vi "Report Status Changes.vi"(5 "Seq Name":string, 6 "Loop Data in":T1, 7 "VolatusAPI":refnum<class "VolatusAPI.lvclass">, 9 "Previous Late":bool, 10 "Previous Duration":i64, 11 "Sequence in":refnum<class "Sequence.lvclass">) -> (4 "Loop Data":T1)   [LabVIEW 2023, in "VolatusSeq.lvlib" / "Sequence.lvclass"]
uses:
  Sequence.lvclass
  Volatus/VolatusAPI/VolatusAPI.lvclass
  Loop Data.ctl
  Volatus/MessageQ/MessageQ.lvclass
  Sequence Time.ctl
  Sequence Status.ctl
  Sequence.lvclass/Sequence.ctl
  Volatus/MessageQ/MessageQ.lvclass/MessageQ.ctl
  VolatusSeq.lvlib
  State/State.lvclass
  VolatusSeqConfig/Debug Flags.ctl
  VolatusSeqConfig/VolatusSeqConfig.lvlib
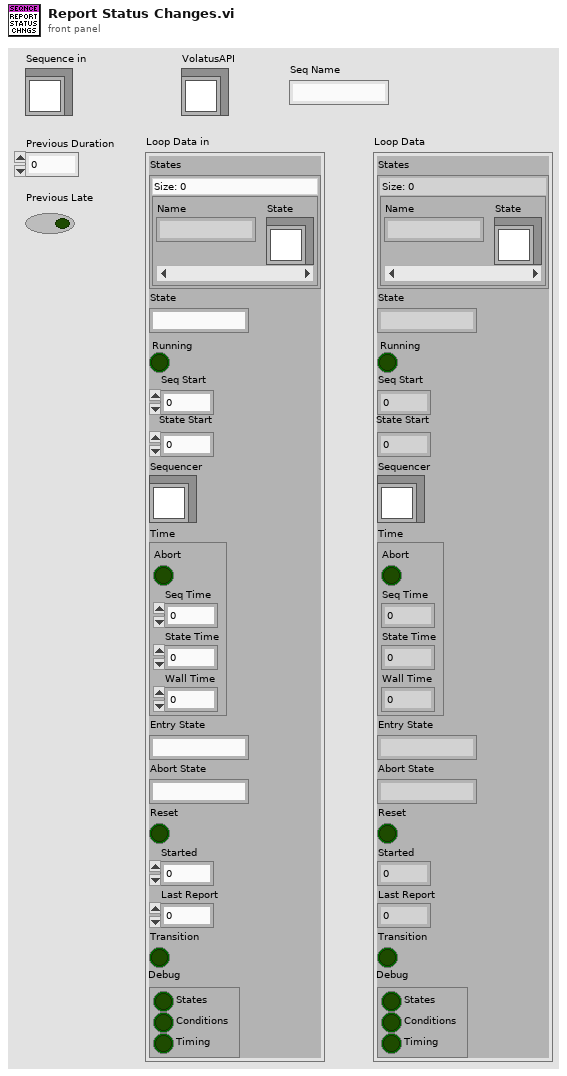
[diagram p1: front panel]
types:
  T1 = typedef "VolatusSeq.lvlib/Sequence.lvclass/Loop Data.ctl" = cluster{"States":map{string, refnum<class "State.lvclass">}, "State":string, "Running":bool, "Seq Start":dbl, "State Start":dbl, "Sequencer":refnum<class "MessageQ.lvclass">, "Time":T2, "Entry State":string, "Abort State":string, "Reset":bool, "Started":dbl, "Last Report":dbl, "Transition":bool, "Debug":T3}
  T2 = typedef "VolatusSeq.lvlib/Sequence Time.ctl" = cluster{"Abort":bool, "Seq Time":dbl, "State Time":dbl, "Wall Time":dbl}
  T3 = typedef "VolatusSeqConfig.lvlib/Debug Flags.ctl" = cluster{"States":bool, "Conditions":bool, "Timing":bool}
  T4 = typedef "VolatusSeq.lvlib/Sequence Status.ctl" = cluster{"Name":string, "State":string, "Time":T2, "Running":bool, "Start Time":dbl, "Previous Duration":i64, "Previous Late":bool}
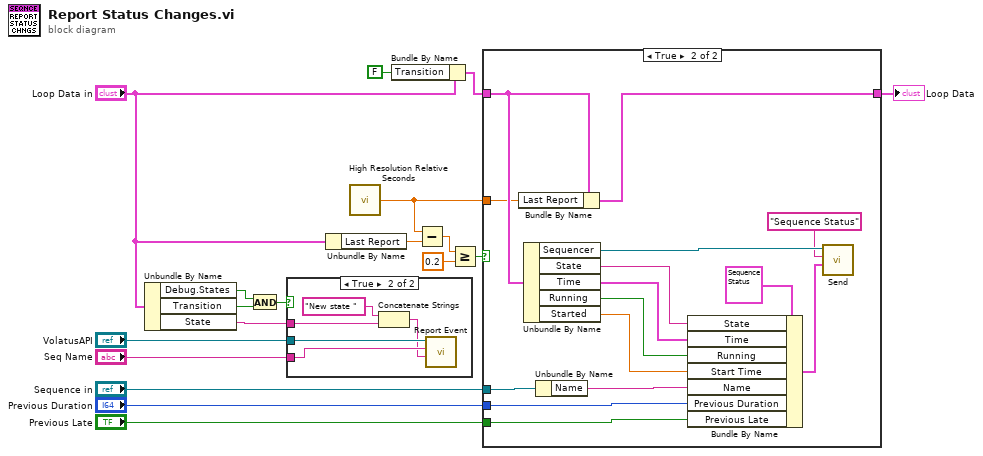
[diagram p0: block diagram]
diagram:
  n1 = Unbundle By Name("Loop Data in") -> ("Debug.States"=w5:bool, "Transition"=w6:bool, "State"=w3:string)
  n2 = And(x=w5, y=w6) -> (x .and. y?=w4:bool)
  n3 = case shown="True" w4 {
    tunnel: w3 -> [_ w20]
    tunnel: "VolatusAPI" -> [_ w23]
    tunnel: "Seq Name" -> [_ w22]
    frame False {
    }
    frame True {
      n4 = Concatenate Strings("New state ", w20) -> (w19:string)
      n5 = call "Report Event.vi"("Message"=w19, "Context"=w22, "VolatusAPI in"=w23) -> ()  [unwired: 7 in, 2 out]
    }
  }
  n6 = Unbundle By Name("Loop Data in") -> ("Last Report"=w15:dbl)
  n7 = call <vilib>:"High Resolution Relative Seconds.vi"() -> ("relative seconds"=w10:dbl)
  n8 = Bundle By Name(cluster="Loop Data in", "Transition"=FALSE) -> (w8:T1)
  n9 = Subtract(x=w10, y=w15) -> (x-y=w14:dbl)
  n10 = Greater Or Equal?(x=w14, y=0.2) -> (x >= y?=w12:bool)
  n11 = case shown="True" w12 {
    tunnel: "Sequence in" -> [_ w39]
    tunnel: "Previous Duration" -> [_ w29]
    tunnel: "Previous Late" -> [_ w28]
    tunnel: w8 -> [w24 w27]
    tunnel: [w24 w26] -> w11
    tunnel: w10 -> [_ w25]
    frame False {
    }
    frame True {
      n12 = Bundle By Name(cluster=w27, "Last Report"=w25) -> (w26:T1)
      n13 = Unbundle By Name(w27) -> ("Sequencer"=w34:refnum<class "MessageQ.lvclass">, "State"=w36:string, "Time"=w35:T2, "Running"=w31:bool, "Started"=w30:dbl)
      n14 = Unbundle By Name(w39) -> ("Name"=w37:string)
      n15 = Bundle By Name(cluster=T4 {"Name"="", "State"="", "Time"={"Abort"=FALSE, "Seq Time"=0.0, "State Time"=0.0, "Wall Time"=0.0}, "Running"=FALSE, "Start Time"=0.0, "Previous Duration"=0, "Previous Late"=FALSE} ("Sequence Status"), "State"=w36, "Time"=w35, "Running"=w31, "Start Time"=w30, "Name"=w37, "Previous Duration"=w29, "Previous Late"=w28) -> (w33:T4)
      n16 = call "Send.vi"("Data"=w33, "ID"="Sequence Status", "MessageQ in"=w34) -> ()  [unwired: 7 in, 2 out]
    }
  }
  "Loop Data" <- w11
